vi "ConvertQTToImageFormat.vi"(1 "Image In":T1 {"Dialogs" format="%.0b"}) -> (0 "image data out":T2)   [LabVIEW 2022 SP3]
uses:
  <vilib>/picture/picture.llb/imagedata.ctl
  <vilib>/addons/RoboLab/ImageProcessing/QTLIB_2595_LV86/QT_Image.ctl
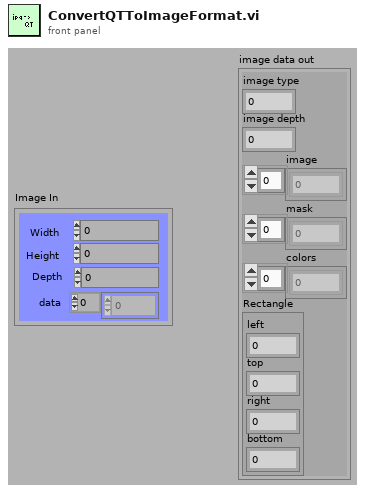
[diagram p1: front panel]
types:
  T1 = typedef "QT_Image.ctl" = cluster{"Width":i32, "Height":i32, "Depth":i32, "data":u8[], "Compressed data":u8[], "Color table":u32[], "Duration":i32, "Options":i32, "Timestamp":i32, "ID":i32, "Reserved":i32, "Dialogs":u32}
  T2 = typedef "imagedata.ctl" = cluster{"image type":i32, "image depth":i32, "image":u8[], "mask":u8[], "colors":u32[], "Rectangle":cluster{"left":i16, "top":i16, "right":i16, "bottom":i16}}
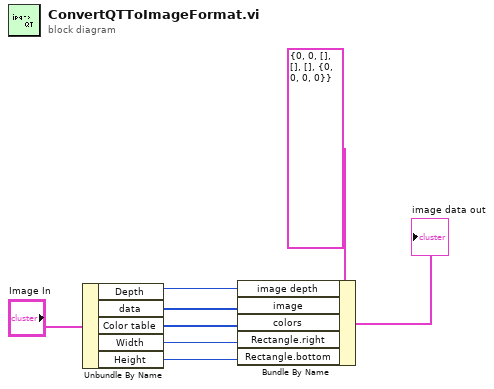
[diagram p0: block diagram]
diagram:
  n1 = Unbundle By Name("Image In") -> ("Depth"=w5:i32, "data"=w4:u8[], "Color table"=w3:u32[], "Width"=w2:i32, "Height"=w1:i32)
  n2 = Bundle By Name(cluster=T2 {"image type"=0, "image depth"=0, "image"=[], "mask"=[], "colors"=[], "Rectangle"={"left"=0, "top"=0, "right"=0, "bottom"=0}} ("image data"), "image depth"=w5, "image"=w4, "colors"=w3, "Rectangle.right"=w2, "Rectangle.bottom"=w1) -> (→"image data out":T2)
